vi "05c-multifunc_external-server.vi"() -> ()   [LabVIEW 2018, in "LV2Julia_examples.lvlib"]
uses:
  LV2Julia_examples.lvlib
  LV2Julia_core/VIs/Server or client state.ctl
  LV2Julia_core/VIs/detailed error info.ctl
  LV2Julia_core/VIs/StackFrame.ctl
  LV2Julia_core/VIs/Commands.ctl
  1e32e5d8-80f1-4661-9552-ce4369739336.vi
  1e32e5d8-80f1-4661-9552-ce4369739336.vi/9833f35b-4200-465e-8f96-465b5dfd780f.vi
  1e32e5d8-80f1-4661-9552-ce4369739336.vi/9833f35b-4200-465e-8f96-465b5dfd780f.vi/094b9caa-5e4a-4df4-8979-1508e6e07af0.vi
  1e32e5d8-80f1-4661-9552-ce4369739336.vi/9833f35b-4200-465e-8f96-465b5dfd780f.vi/3706e0cb-2f7c-4b76-ab31-a3ce7c9366b6.vi
  1e32e5d8-80f1-4661-9552-ce4369739336.vi/9833f35b-4200-465e-8f96-465b5dfd780f.vi/90c53667-b803-4f95-a63e-2024f070532c.vi
  LV2Julia_core/VIs/jl-scripts path.vi
  LV2Julia_core/VIs/check ID validity.vi
  LV2Julia_core/VIs/bindata_descr to JSON.vi
  LV2Julia_core/VIs/check cluster field names.vi
  LV2Julia_core/VIs/concat JSON.vi
  LV2Julia_core/VIs/build request.vi
  LV2Julia_core/VIs/Parse server response.vi
  LV2Julia_core/VIs/log jl exceptions.vi
  LV2Julia_core/LV2Julia_core.lvlib
panel:
  in  "execution control pages":enum32{"Start", "go - test"}(tab)
  in  "go":bool caption="go (Julia Server started externally)"
  in  "Start with Julia":bool caption="Start Julia Server and go"
  in  "ZMQ endpoint":string="tcp://127.0.0.1:5555"
  in  "stop this VI only":bool
  in  "stop both this VI and Julia Server":bool
  in  "operation":T1(radio)
  in  "operands":cluster{"x":dbl, "y":dbl}={"x"=2.0, "y"=2.0}
  in  "next":bool
  out "x+y":dbl=nan
  out "detailed error info":T2
  out "current error":errorcluster
  out "final error":errorcluster
  out "short err code":u8
  out "call duration (ms)":dbl format="%#.2f"
  out "ZMQ timeout":bool
  out "Julia script file path":path
  out "temporary script path":path
  out "Jl Server state":T4
  # "tcp://127.0.0.1:5555 \nfor local Julia Server\n\nFor a Julia Server running on a separate computer,  you probably must use an IPv4 address in numeric form (not a DNS name) - see https://stackoverflow.com/questions/6024003/why-doesnt-zeromq-work-on-localhost.\n\nFor instructions how to properly start the corresponding Julia script, see \n05-on_external_server.jl file in the jl-scripts folder.\n\nThe ZMQ endpoint control only used if Julia Server is not being started by this VI."
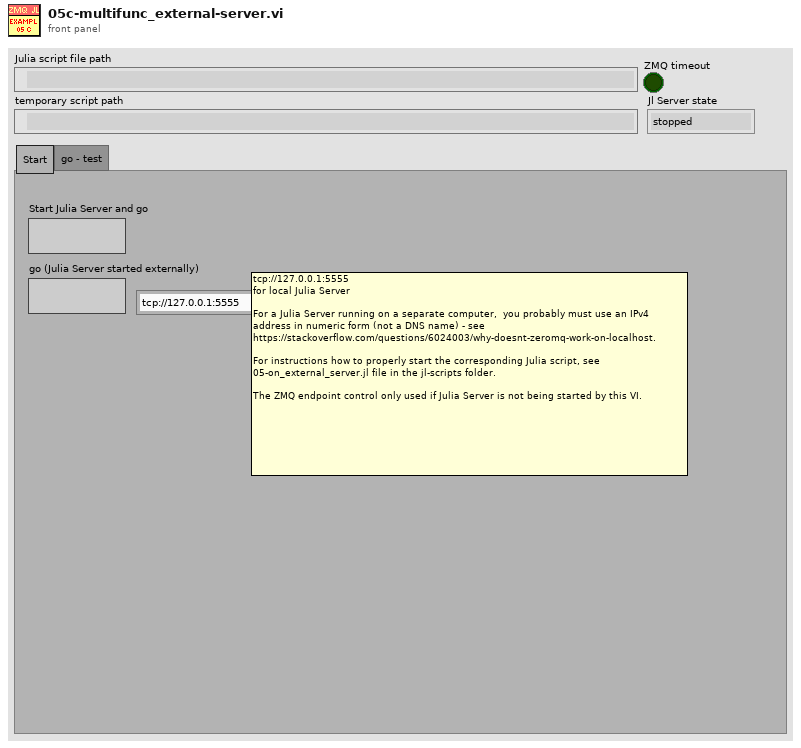
[diagram p1: front panel]
types:
  T1 = enum32{"add", "subtract", "multiply", "divide", "conquer"}
  T2 = typedef "LV2Julia_core.lvlib/detailed error info.ctl" = cluster{"exception_or_info":string, "trace":T3[]}
  T3 = typedef "LV2Julia_core.lvlib/StackFrame.ctl" = cluster{"frame_summary":string, "func":string, "linfo":string, "file":string, "line":i32, "pointer":u64, "from_c":bool, "inlined":bool}
  T4 = typedef "LV2Julia_core.lvlib/Server or client state.ctl" = enum16{"stopped", "running", "unknown"}
  T5 = typedef "LV2Julia_core.lvlib/Commands.ctl" = enum16{"Start Jl-server & Init LV-client", "Send request & Get response ", "Stop Jl-server & Cleanup LV-client", "Cleanup LV-client", "Start Jl-server", "Stop Jl-server", "Init LV-Client", "Cleanup LV-Client", "(not allowed)", "Set LV Client state", "Set Jl Server state", "set ZMQ timeout", "read ZMQ timeout", "read-out state"}
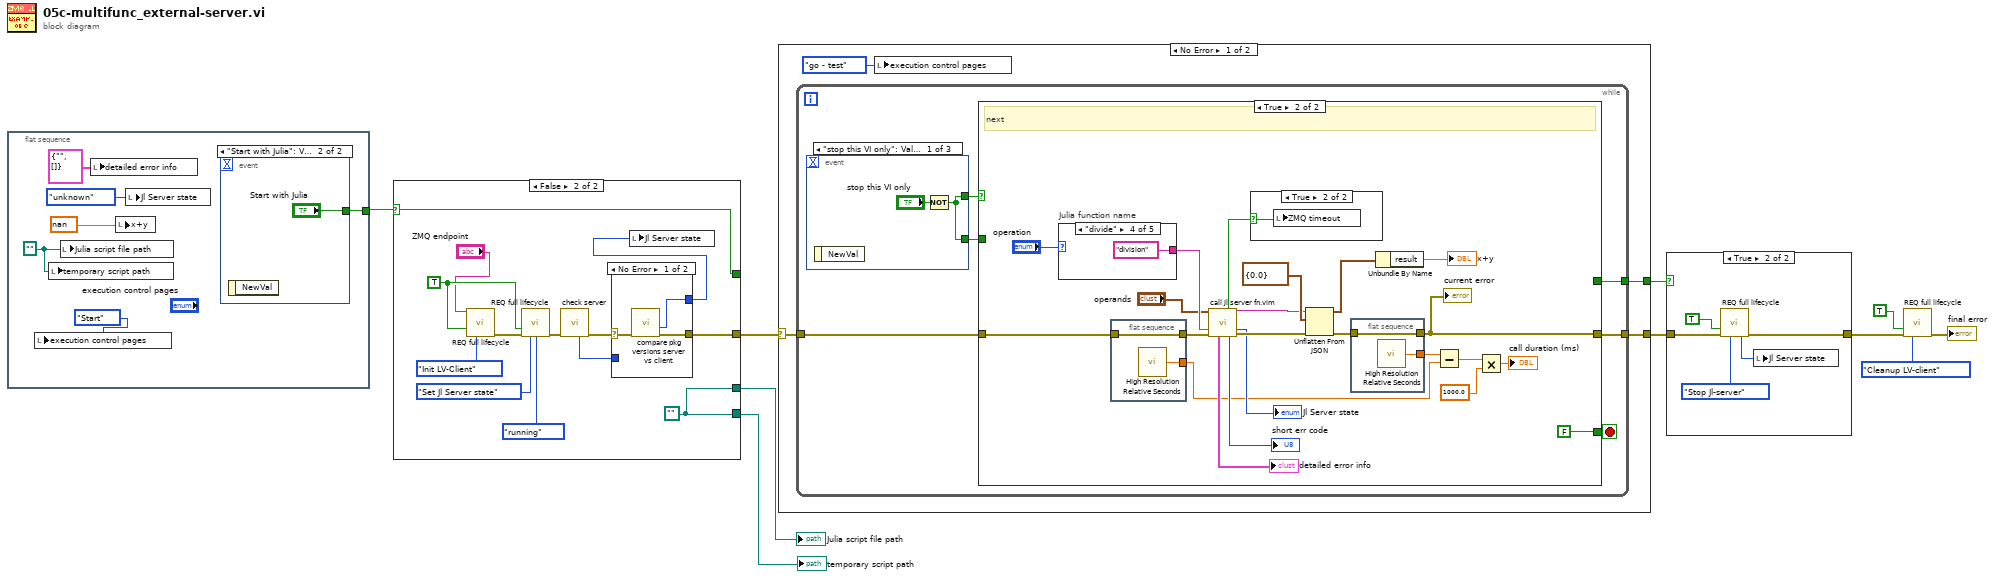
[diagram p0: block diagram]
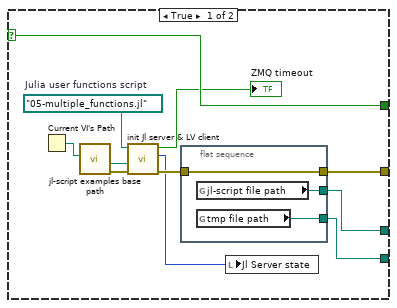
[diagram p3: hidden frame]
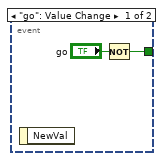
[diagram p5: hidden frame]
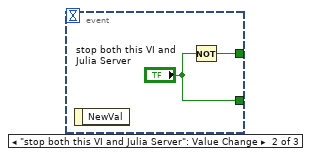
[diagram p6: hidden frame]
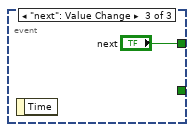
[diagram p7: hidden frame]
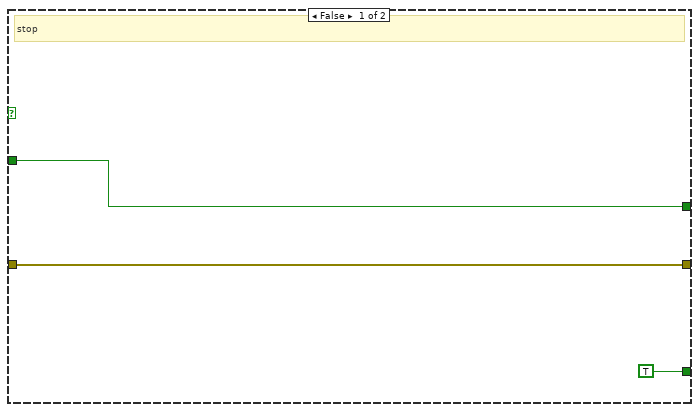
[diagram p8: hidden frame]
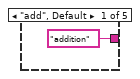
[diagram p9: hidden frame]
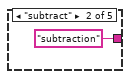
[diagram p10: hidden frame]
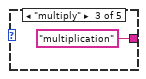
[diagram p11: hidden frame]
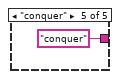
[diagram p12: hidden frame]
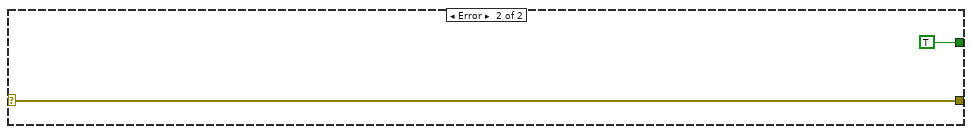
[diagram p14: hidden frame]
diagram:
  n1 = flat-sequence {
    tunnel: [w11] -> w3
    frame #0 {
      w13 = path ""
      n2 = local write "execution control pages"(enum32{"Start", "go - test"}."Start" ("execution control pages")) -> ()
      n3 = local write "temporary script path"(w13) -> ()
      n4 = local write "Julia script file path"(w13) -> ()
      n5 = local write "detailed error info"(T2 {"exception_or_info"="", "trace"=[]} ("detailed error info")) -> ()
      n6 = local write "x+y"(nan ("Server response")) -> ()
      n7 = local write "Jl Server state"(Server_or_client_state."unknown" ("Jl Server state out")) -> ()
      n8 = event shown="[1] \"Start with Julia\": Value Change" {
        selector: _ -> [_ _]
        dyn-events: _ -> [_ _]
        timeout: _ -> [_ _]
        tunnel: [w17 "Start with Julia"] -> w11
        event "go": Value Change {
          n9 = event-data() -> ()  [unwired: 1 in, 1 out]
          n10 = Not(x="go") -> (.not. x?=w17:bool)
        }
        event "Start with Julia": Value Change {
          n11 = event-data() -> ()  [unwired: 1 in, 1 out]
        }
      }
    }
  }
  n12 = case shown="False" w3 {
    selector: w3 -> [w30 w42]
    tunnel: [w29 w37] -> w6
    tunnel: [w30 w42] -> _
    tunnel: [w28 w39] -> w4
    tunnel: [w27 w39] -> w5
    frame True {
      w21 = path "05-multiple_functions.jl"  # Julia user functions script
      n13 = Current VI's Path() -> (path=w25:path)
      n14 = call "jl-script examples base path.vi"("calling example VI path"=w25) -> ("error out"=w24:errorcluster, "jl-script-examples base path"=w23:path)  [unwired: 9 in]
      n15 = call "init Jl server & LV client.vi"("error in (no error)"=w24, "Base path (not a path)"=w23, "Julia user functions script"=w21) -> ("error out"=w26:errorcluster, "Jl Server state out"=w22:T4, "timeout?"=→"ZMQ timeout":bool)  [unwired: 6 in]
      n16 = flat-sequence {
        tunnel: [w33] -> w29
        tunnel: w26 -> [w33]
        tunnel: [w32] -> w28
        tunnel: [w31] -> w27
        frame #0 {
          n17 = global read "jl-scripts path.vi" "jl-script file path"() -> (w32:path)
          n18 = global read "jl-scripts path.vi" "tmp file path"() -> (w31:path)
        }
      }
      n19 = local write "Jl Server state"(w22) -> ()
    }
    frame False {
      w39 = path ""
      w44 = TRUE ("Force command")
      n20 = call "REQ full lifecycle.vi"("ZMQ endpoint"="ZMQ endpoint", "Force command"=w44, "command"=Commands."Init LV-Client") -> ("error out"=w41:errorcluster)  [unwired: 6 in, 6 out]
      n21 = call "REQ full lifecycle.vi"("Force command"=w44, "error in"=w41, "command"=Commands."Set Jl Server state", "Jl Server state in"=Server_or_client_state."running") -> ("error out"=w40:errorcluster)  [unwired: 5 in, 6 out]
      n22 = call "check server.vi"("error in"=w40) -> ("error out"=w38:errorcluster, "Jl Server state out"=w36:T4)  [unwired: 6 in, 3 out]
      n23 = case shown="No Error" w38 {
        selector: w38 -> [w49 w51]
        tunnel: [w48 w51] -> w37
        tunnel: [w47 w50] -> w34
        tunnel: w36 -> [_ w50]
        frame No Error {
          n24 = call "compare pkg versions server vs client.vi"("error in (no error)"=w49) -> ("error out"=w48:errorcluster, "Jl Server state out"=w47:T4)  [unwired: 4 in, 5 out]
        }
        frame Error {
        }
      }
      n25 = local write "Jl Server state"(w34) -> ()
    }
  }
  "temporary script path" <- w5
  "Julia script file path" <- w4
  n26 = case shown="No Error" w6 {
    selector: w6 -> [w54 w103]
    tunnel: [w55 w103] -> w10
    tunnel: [w52 TRUE ("stop both this VI and Julia Server")] -> w1
    frame No Error {
      n27 = while {
        tunnel: w54 -> [w60]
        tunnel: [w61] -> w55
        tunnel: [w56] -> w52
        stop <- w58 stop-if-true
        n28 = event shown="[0] \"stop this VI only\": Value Change" {
          selector: _ -> [_ _ _]
          dyn-events: _ -> [_ _ _]
          timeout: _ -> [_ _ _]
          tunnel: [w62 w65 "next"] -> w59
          tunnel: [w62 "stop both this VI and Julia Server" _] -> w57
          event "stop this VI only": Value Change {
            n29 = event-data() -> ()  [unwired: 1 in, 1 out]
            n30 = Not(x="stop this VI only") -> (.not. x?=w62:bool)
          }
          event "stop both this VI and Julia Server": Value Change {
            n31 = event-data() -> ()  [unwired: 1 in, 1 out]
            n32 = Not(x="stop both this VI and Julia Server") -> (.not. x?=w65:bool)
          }
          event "next": Value Change {
            n33 = event-data() -> ()  [unwired: 1 in, 1 out]
          }
        }
        n34 = case shown="True" w59 {
          tunnel: [w69 w70] -> w61
          tunnel: w60 -> [w69 w73]
          tunnel: [TRUE ("stop this VI only") FALSE ("stop this VI only")] -> w58
          tunnel: w57 -> [w67 _]
          tunnel: [w67 _] -> w56
          frame False {
            # "stop"
          }
          frame True {
            # "next"
            n35 = case "Julia function name" shown="\"divide\"" "operation" {
              tunnel: ["addition" "subtraction" "multiplication" "division" "conquer"] -> w85
              frame "add", Default {
              }
              frame "subtract" {
              }
              frame "multiply" {
              }
              frame "divide" {
              }
              frame "conquer" {
              }
            }
            n36 = flat-sequence {
              tunnel: [w95] -> w76
              tunnel: [w94] -> w72
              tunnel: w73 -> [w94]
              frame #0 {
                n37 = call <vilib>:"High Resolution Relative Seconds.vi"() -> ("relative seconds"=w95:dbl)
              }
            }
            n38 = call "call Jl server fn.vim"("Arguments 1"="operands", "fun2call"=w85, "error in (no error)"=w72) -> ("timeout?"=w82:bool, "JSON received"=w81:string, "Jl Server state out"=→"Jl Server state":T4, "detailed error info"=→"detailed error info":T2, "return code"=→"short err code":u8, "error out"=w86:errorcluster)  [unwired: 6 in, 1 out]
            n39 = case shown="True" w82 {
              selector: w82 -> [_ w101]
              frame False {
              }
              frame True {
                n40 = local write "ZMQ timeout"(w101) -> ()
              }
            }
            n41 = Unflatten From JSON(JSON string=w81, type and defaults=cluster{"result":dbl} {"result"=0.0} ("parsed response"), error in (no error)=w86) -> (value=w90:cluster{"result":dbl}, error out=w71:errorcluster)  [unwired: 4 in]
            n42 = flat-sequence {
              tunnel: [w93] -> w75
              tunnel: [w92] -> w70
              tunnel: w71 -> [w92]
              frame #0 {
                n43 = call <vilib>:"High Resolution Relative Seconds.vi"() -> ("relative seconds"=w93:dbl)
              }
            }
            n44 = Unbundle By Name(w90) -> ("result"=→"x+y":dbl)
            n45 = Subtract(x=w75, y=w76) -> (x-y=w77:dbl)
            n46 = Multiply(x=w77, y=1000.0) -> (x*y=→"call duration (ms)":dbl)
            "current error" <- w70
          }
        }
      }
      n47 = local write "execution control pages"(enum32{"Start", "go - test"}."go - test" ("execution control pages")) -> ()
    }
    frame Error {
    }
  }
  n48 = case shown="True" w1 {
    tunnel: w10 -> [w104 w109]
    tunnel: [w104 w107] -> w9
    frame False {
    }
    frame True {
      n49 = call "REQ full lifecycle.vi"("Force command"=TRUE, "error in"=w109, "command"=Commands."Stop Jl-server") -> ("Jl Server state out"=w106:T4, "error out"=w107:errorcluster)  [unwired: 6 in, 5 out]
      n50 = local write "Jl Server state"(w106) -> ()
    }
  }
  n51 = call "REQ full lifecycle.vi"("Force command"=TRUE, "error in"=w9, "command"=Commands."Cleanup LV-client") -> ("error out"=→"final error":errorcluster)  [unwired: 6 in, 6 out]
